vi "Calculate_ROI_matrix.vi"(8 "error in (no error)":errorcluster, 10 "PicamROI":T1) -> (0 "error out":errorcluster, 1 "Columns (pixels)":i32, 2 "Rows (pixels)":i32)   [LabVIEW 2014, in "PICam.lvlib"]
uses:
  PICam.lvlib
  Ctrls/PicamROI.ctl
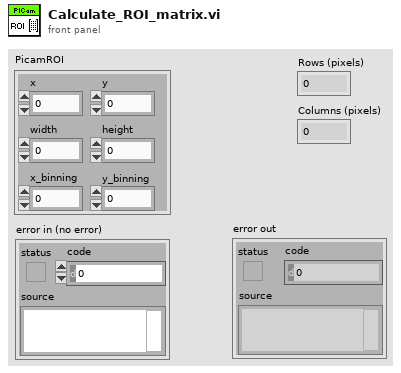
[diagram p1: front panel]
types:
  T1 = typedef "PICam.lvlib/PicamROI.ctl" = cluster{"x":i32, "width":i32, "x_binning":i32, "y":i32, "height":i32, "y_binning":i32}
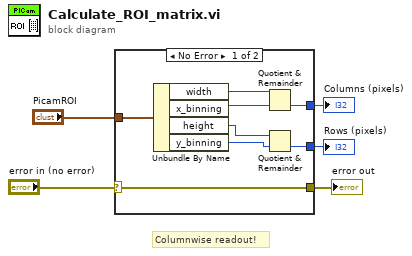
[diagram p0: block diagram]
diagram:
  # "Columnwise readout!"
  n1 = case shown="No Error" "error in (no error)" {
    selector: "error in (no error)" -> [w13 w14]
    tunnel: [w13 w14] -> w4
    tunnel: "PicamROI" -> [w12 _]
    tunnel: [w7 _] -> w2
    tunnel: [w6 _] -> w1
    frame No Error {
      n2 = Unbundle By Name(w12) -> ("width"=w11:i32, "x_binning"=w10:i32, "height"=w9:i32, "y_binning"=w8:i32)
      n3 = Quotient & Remainder(x=w11, y=w10) -> (floor(x/y)=w7:i32)  [unwired: 1 out]
      n4 = Quotient & Remainder(x=w9, y=w8) -> (floor(x/y)=w6:i32)  [unwired: 1 out]
    }
    frame Error {
    }
  }
  "error out" <- w4
  "Columns (pixels)" <- w2
  "Rows (pixels)" <- w1
